vi "staticvi.vi"   [LabVIEW 2014]
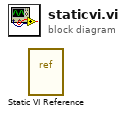
[diagram p0: block diagram]
diagram:
  n1 = vi-ref "Static VI Reference"() -> ()  [unwired: 1 out]
